vi "DeCoF real set.vi"(4 "error in":errorcluster, 5 "value":dbl, 6 "param-name":string, 7 "Conncection ID in":T1) -> (0 "error out":errorcluster, 3 "Conncection ID out":T1)   [LabVIEW 2013]
uses:
  subVIs/DeCoF connection.ctl
panel:
  out "answer string":string
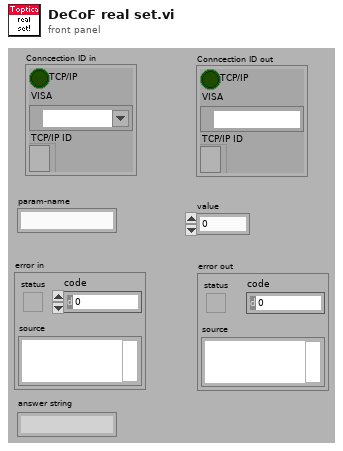
[diagram p1: front panel]
types:
  T1 = typedef "DeCoF connection.ctl" = cluster{"TCP/IP":bool, "VISA":refnum<visa-resource-name>, "TCP/IP ID":refnum<k5>}
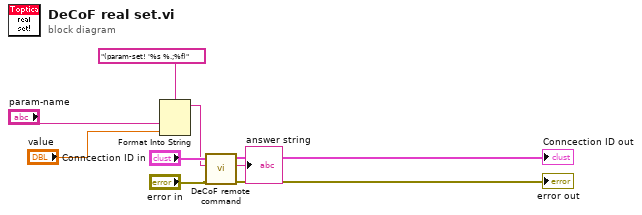
[diagram p0: block diagram]
diagram:
  n1 = Format Into String(format string="(param-set! '%s %.;%f)", "param-name", "value") -> (resulting string=w4:string)  [unwired: 2 in, 1 out]
  n2 = call "DeCoF remote command.vi"("error in (no error)"="error in", "command"=w4, "Conncection ID in"="Conncection ID in") -> ("error out"=→"error out":errorcluster, "answer string"=→"answer string":string, "Conncection ID out"=→"Conncection ID out":T1)  [unwired: 2 in, 2 out]
